vi "test circle.vi"() -> ()   [LabVIEW 2010]
uses:
  polar tracking settings.ctl
panel:
  out "output cluster":T1={"scan radius"=0, "2^16/lines per revolution"=1394, "gx"=0.0, "rtw"=0.0, "lines per revolution"=47, "vel diff"=0.0}
  out "prod xy":i32
  in  "x-y phase shift (*2^16/2*pi)":u16=16384
  out "y":i16[](array[numeric])
  out "x":i16[](array[numeric])
  out "XY Graph":cluster{i16[], i16[]}(graph)
  out "line num":u8[](array[numeric])
  in  "tracking settings":T1={"scan radius"=1000, "2^16/lines per revolution"=1024, "gx"=0.0, "rtw"=0.0, "lines per revolution"=64, "vel diff"=0.0}
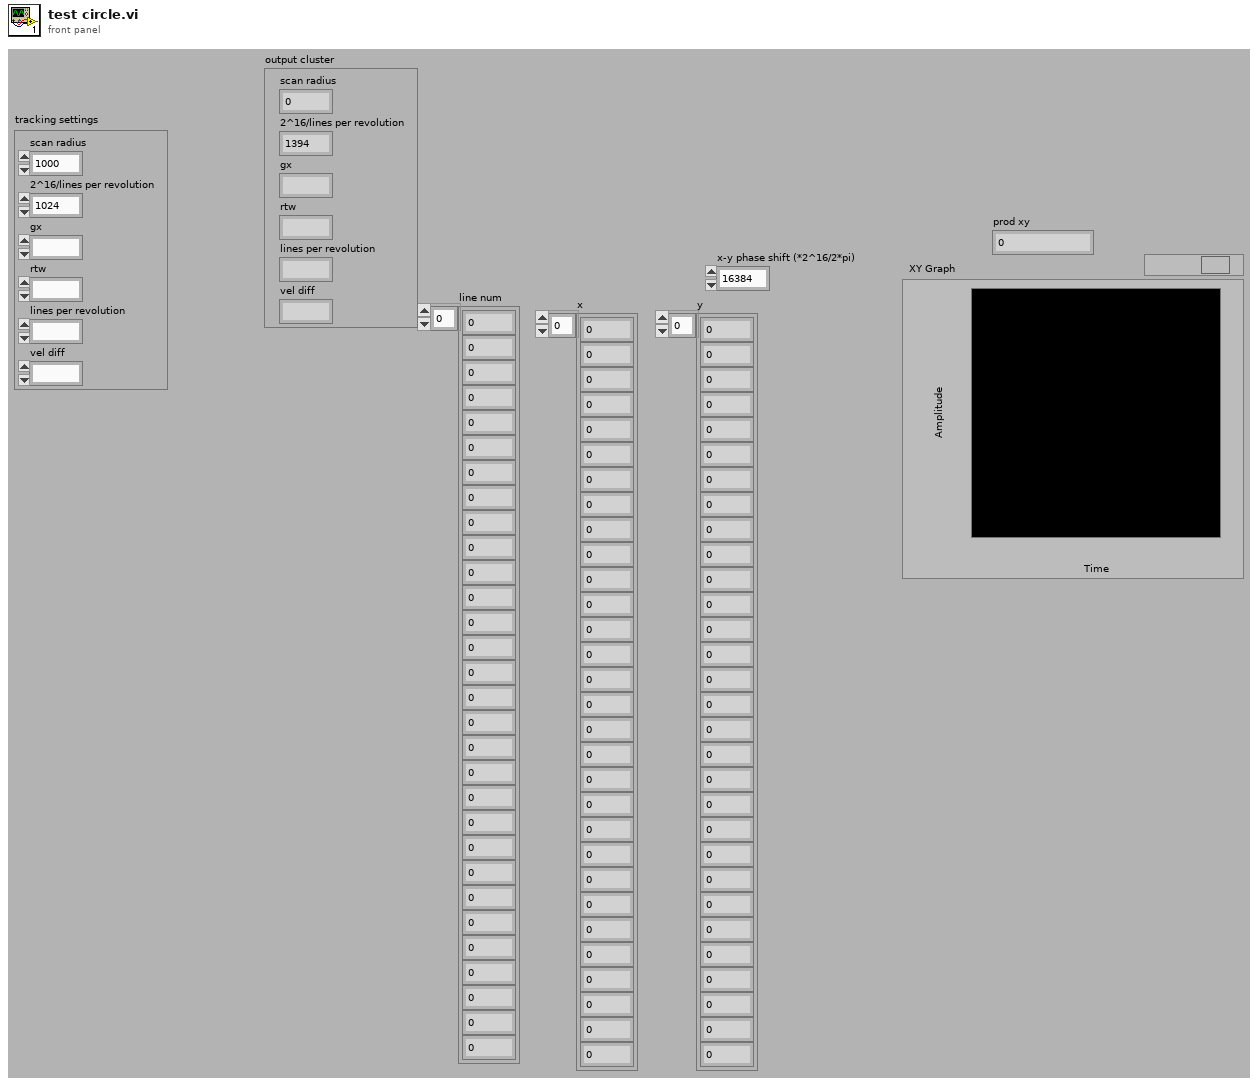
[diagram p1: front panel]
types:
  T1 = typedef "polar tracking settings.ctl" = cluster{"scan radius":u16, "2^16/lines per revolution":u16, "gx":fxp<+,16,8>, "rtw":fxp<+,16,26>, "lines per revolution":u8, "vel diff":fxp<+,24,-22>}
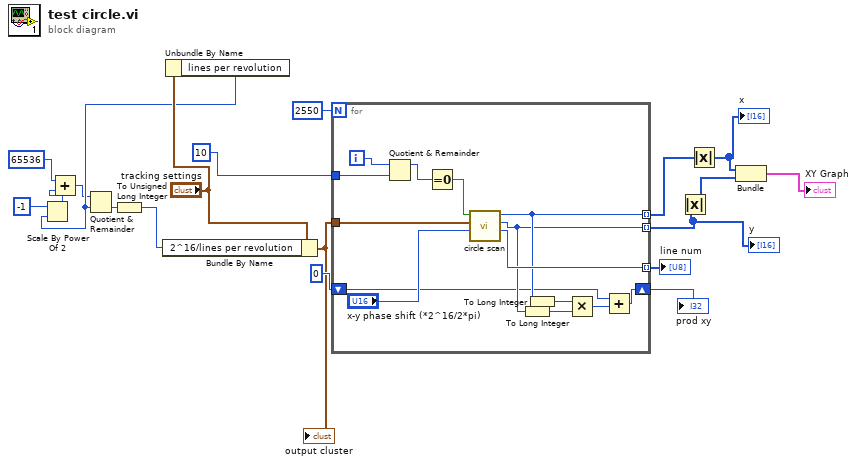
[diagram p0: block diagram]
diagram:
  n1 = Unbundle By Name("tracking settings") -> ("lines per revolution"=w8:u8)
  n2 = Scale By Power Of 2(n=i16 -1, x=w8) -> (x*2^n=w7:u8)
  n3 = Add(x=u32 65536, y=w7) -> (x+y=w6:u32)
  n4 = Quotient & Remainder(x=w6, y=w8) -> (floor(x/y)=w11:u32)  [unwired: 1 out]
  n5 = To Unsigned Long Integer(number=w11) -> (unsigned 32bit integer=w5:u32)
  n6 = Bundle By Name(cluster="tracking settings", "2^16/lines per revolution"=w5) -> (w3:T1)
  "output cluster" <- w3
  n7 = for {
    N: 2550 -> [_]
    tunnel: [w29] -> w17 mode=indexing
    tunnel: [w28] -> w16 mode=indexing
    tunnel: [w33] -> w19 mode=indexing
    shift-right: [w24] -> w14
    shift-left: 0 -> [w23]
    tunnel: w3 -> [w22]
    tunnel: 10 ("y") -> [w21]
    i -> [w31]
    n8 = Quotient & Remainder(x=w31, y=w21) -> (x-y*floor(x/y)=w30:i32)  [unwired: 1 out]
    n9 = Equal To 0?(x=w30) -> (x = 0?=w20:bool)
    n10 = call "circle scan.vi"("x-y phase shift (*2^16/2*pi)"="x-y phase shift (*2^16/2*pi)", "tracking settings"=w22, "new line"=w20) -> ("line counter"=w33:u8, "y value"=w28:i16, "x value"=w29:i16)  [unwired: 6 in]
    n11 = To Long Integer(number=w28) -> (32bit integer=w26:i32)
    n12 = To Long Integer(number=w29) -> (32bit integer=w27:i32)
    n13 = Multiply(x=w27, y=w26) -> (x*y=w25:i32)
    n14 = Add(x=w23, y=w25) -> (x+y=w24:i32)
  }
  "line num" <- w19
  "y" <- w16
  "prod xy" <- w14
  n15 = Absolute Value(x=w16) -> (abs(x)=w2:i16[])
  n16 = Absolute Value(x=w17) -> (abs(x)=w1:i16[])
  "x" <- w1
  n17 = Bundle(w1, w2) -> (→"XY Graph":cluster{i16[], i16[]})  [unwired: 1 in]
